vi "Read Input Filter.vi"(8 "error in (no error)":errorcluster, 11 "SD Module in":refnum<class "SD Module.lvclass">) -> (0 "error out":errorcluster, 2 "Input Filter":u32(ring)=128 items=["1 us"=0, "16 us"=1, "256 us"=2, "4096 us"=3, "Disabled"=128], 3 "SD Module out":refnum<class "SD Module.lvclass">)   [LabVIEW 2019, in "Modules.lvlib" / "SD Module.lvclass"]
uses:
  SD Module.lvclass
  SD Module.lvclass/SD Module.ctl
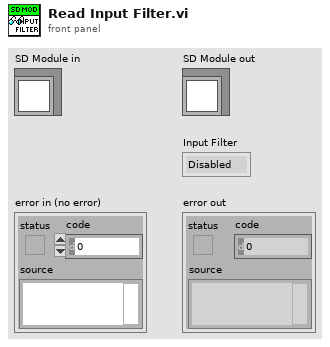
[diagram p1: front panel]
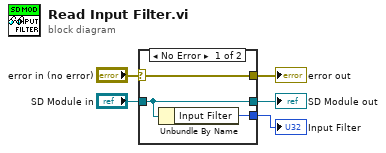
[diagram p0: block diagram]
diagram:
  n1 = case shown="No Error" "error in (no error)" {
    selector: "error in (no error)" -> [w8 w9]
    tunnel: [w8 w9] -> w4
    tunnel: [w7 w10] -> w2
    tunnel: "SD Module in" -> [w7 w10]
    tunnel: [w6 _] -> w1
    frame No Error {
      n2 = Unbundle By Name(w7) -> ("Input Filter"=w6:u32)
    }
    frame Error {
    }
  }
  "error out" <- w4
  "SD Module out" <- w2
  "Input Filter" <- w1
